vi "Global.vi"() -> ()   [LabVIEW 2013, in "AIT 1553 Custom Device.lvlib"]
uses:
  AIT 1553 Custom Device.lvlib
panel:
  in  "Board Index":string="Board Index"
  in  "Licensed?":string="Licensed?"
  in  "RTReadRate":string="BMReadRate"
  in  "Bus Monitor Parm Page GUID":string="11250030-7C42-42CF-BB8B-798981AF63E1"
  in  "Bus Monitor Msg Page GUID":string="ECF4EF81-B0E5-4D2A-BF1C-47416AD3A19C"
  in  "Remote Terminal Parm Page GUID":string="11250030-7C42-42CF-BB8B-798981AF63E1"
  in  "Remote Terminal Msg Page GUID":string="ECF4EF81-B0E5-4D2A-BF1C-47416AD3A19C"
  in  "Default Word":string="Default Word"
  in  "First Word":string="First Word"
  in  "Default Message Buffer Data":string="Default Message Buffer Data"
  in  "Message Buffer ID":string="Message Buffer ID"
  in  "RT Sub Address":string="RT Sub Address"
  in  "RT Address":string="RT Address"
  in  "Tx-Rx":string="Tx-Rx"
  in  "Message":string="Message"
  in  "Bus4Enabled":string="Bus4Enabled"
  in  "Bus3Enabled":string="Bus3Enabled"
  in  "Bus2Enabled":string="Bus2Enabled"
  in  "Bus1Enabled":string="Bus1Enabled"
  in  "RTName":string="Remote Terminals"
  in  "BMReadRate":string="BMReadRate"
  in  "BMName":string="Bus Monitor"
  in  "Bus Controller Frame Page GUID":string="5F3A029A-3543-4F73-90C9-3405822BB34E"
  in  "Bus Controller Acyclic Page GUID":string="932CED9F-0945-4D52-A2BE-3AE869EDF67E"
  in  "Bus Controller Parm Page GUID":string="11250030-7C42-42CF-BB8B-798981AF63E1"
  in  "Bus Controller Msg Page GUID":string="ECF4EF81-B0E5-4D2A-BF1C-47416AD3A19C"
  in  "BCParmName":string="BCMsgName"
  in  "BCMsgName":string="BCMsgName"
  in  "BCReadRate":string="BCReadRate"
  in  "Remote Termial Page GUID":string="FF657A95-E92F-49B2-B647-7C517829BFDA"
  in  "Bus Monitor Page GUID":string="690BD4EE-A4BC-46E2-821B-3839E087B4DA"
  in  "Bus Controller Page GUID":string="AD368ECC-83F2-4839-B428-F6389CBFB7B3"
  in  "Bus Page GUID":string="BC139571-F945-4F35-A44F-DE66E866FF2F"
  in  "BCEnabled":string="BCEnabled"
  in  "BCName":string="Bus Controller"
  in  "BusNumber":string="BusNumber"
  in  "BusName":string="BusName"
  in  "LicenseKey":string="LicenseKey"
  in  "AppLicense?":string="AppLicense?"
  in  "ScaleOffset":string="ScaleOffset"
  in  "ScaleFac":string="ScaleFac"
  in  "Signed?":string="Signed?"
  in  "DBHash":string="DBHash"
  in  "MainDisabled":string="D875045B-F708-417A-8922-E756FC4B70ED"
  in  "MainEnabled":string="9F0087A5-0D3D-41AC-84E7-59462FEFDFC4"
  in  "Static Chan GUID":string="D9567732-A0D4-4249-9D7D-90741D022DA7"
  in  "Default Value":string="Default Value"
  in  "Serial#":string="Serial#"
  in  "Status Section GUID":string="2ECB6C91-3CC4-4FDF-AD6F-FA2D8CDB197F"
  in  "Num Bits":string="Num Bits"
  in  "Win File Path":string="Win File Path"
  in  "Start Bit":string="Start Bit"
  # "Main Page Items"
  # "Bus Page Items"
  # "BC Page Items"
  # "BC Msg Page Items"
  # "BC Parameter Page Items"
  # "Section for Acyclic"
  # "Load/Referesh Database"
  # "BM Page Items"
  # "Old"
  # "New"
  # "Run Time Menu Item - Separator"
  # "7755077A-1485-13A6-5674A23FB86277FF"
  # "C4F6D306-C3D2-477F-8B0F-4F0FF7C0D36D"
  # "Add Bus Function"
  # "Run Time Menu Item - Disable"
  # "24B063C9-F831-AFAE-44CD-E299CAF12166"
  # "4BD42C26-0AA1-42C2-86E5-FB8DBEEA74AE"
  # "RT Page Items"
  # "Main Enabled"
  # "961BA415-D612-25DB-1EE4-93AC9399C9B8"
  # "9F0087A5-0D3D-41AC-84E7-59462FEFDFC4"
  # "D875045B-F708-417A-8922-E756FC4B70ED"
  # "Main Disabled"
  # "C84F327B-5F00-A71A-4A47-A7C0FE0BF79D"
  # "Static Chan"
  # "D9567732-A0D4-4249-9D7D-90741D022DA7"
  # "620FF26C-B46F-A798-9FE7-99E7CBCC898B"
  # "Status Section"
  # "40A8AAAE-6936-1961-F317-B9DADC611A49"
  # "2ECB6C91-3CC4-4FDF-AD6F-FA2D8CDB197F"
  # "GUIDS"
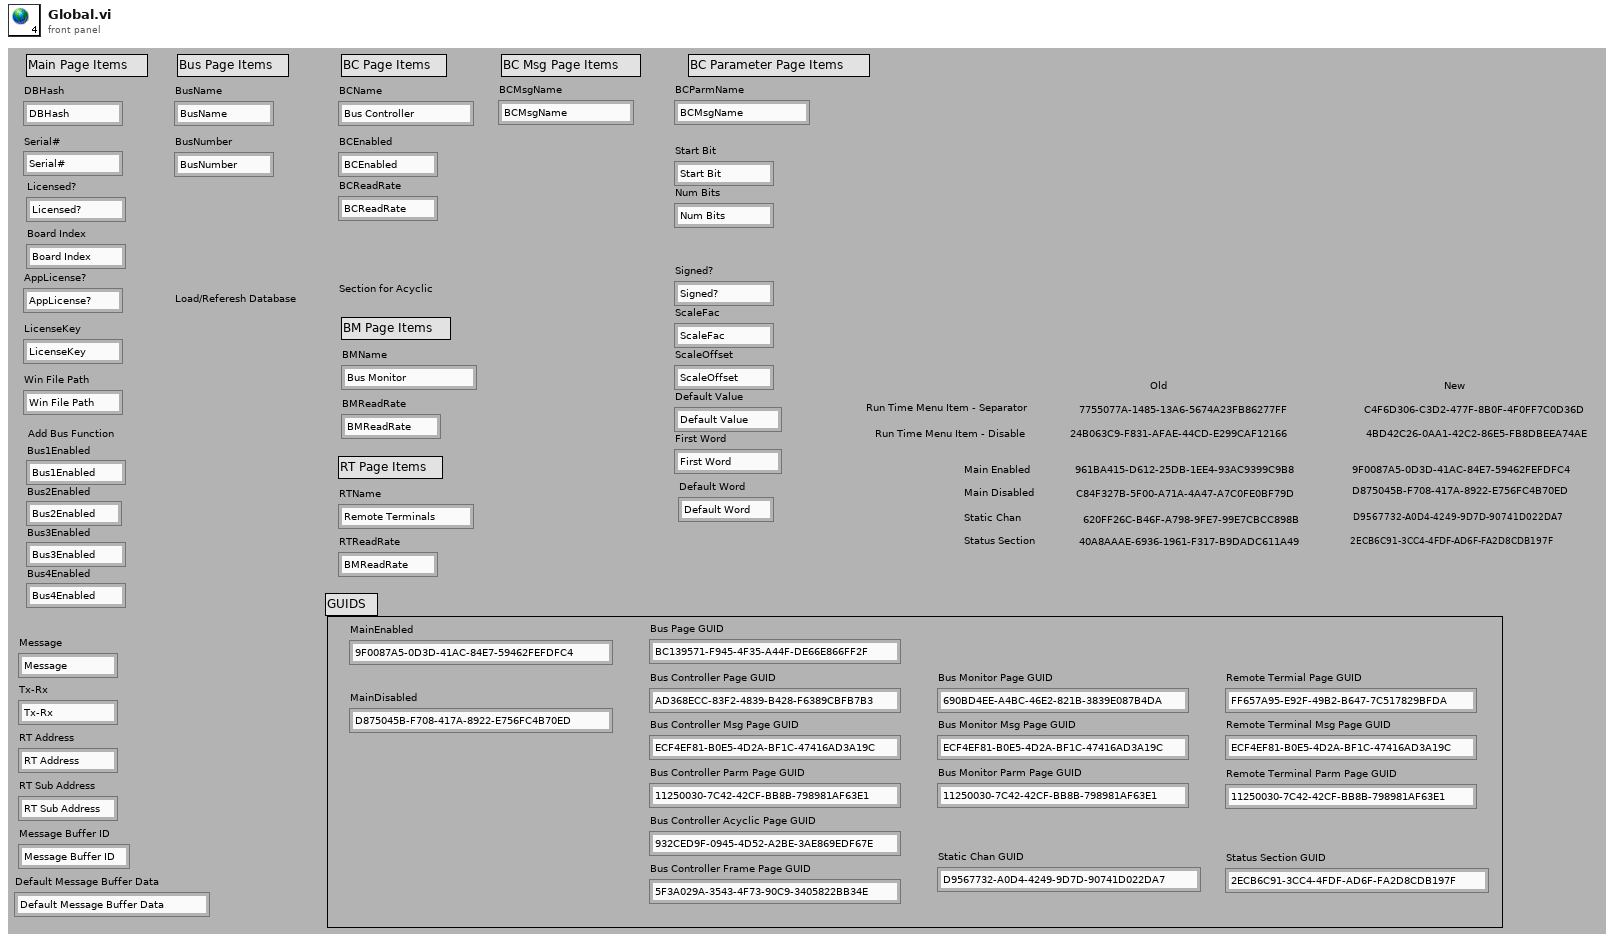
[diagram p1: front panel]
diagram:
